vi "Stack Header (SubVI).vi"(7 "Image Size":T1={"Height"=3072, "Width"=3072}) -> (3 "Complete Header":u8[](array[numeric]))   [LabVIEW 2015]
uses:
  Controls (HOST)/Image Size.ctl
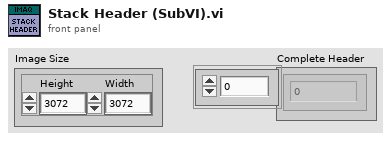
[diagram p1: front panel]
types:
  T1 = typedef "Image Size.ctl" = cluster{"Height":u16, "Width":u16}
  T2 = enum16{"big-endian, network order", "native, host order", "little-endian"}
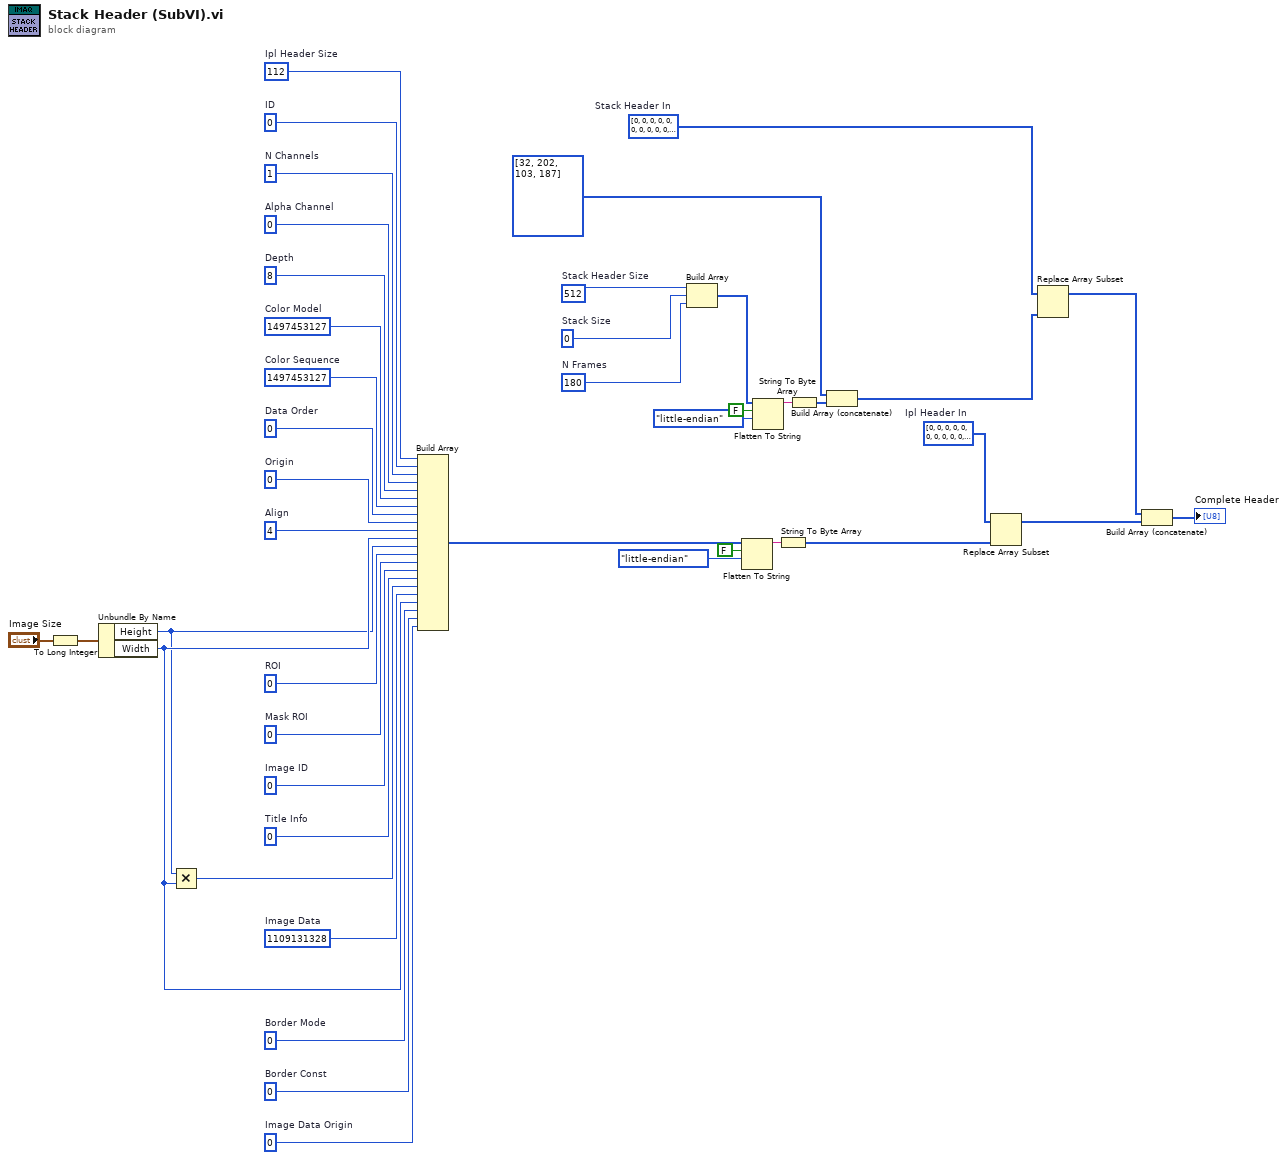
[diagram p0: block diagram]
diagram:
  w10 = 180  # N Frames
  w11 = 0  # Stack Size
  w12 = 512  # Stack Header Size
  w2 = u8[] [0, 0, 0, 0, 0, 0, 0, 0, 0, 0, 0, 0, 0, 0, 0, 0, 0, 0, 0, 0, 0, 0, 0, 0, 0, 0, 0, 0, 0, 0, 0, 0, 0, 0, 0, 0, 0, 0, 0, 0, 0, 0, 0, 0, 0, 0, 0, 0, 0, 0, 0, 0, 0, 0, 0, 0, 0, 0, 0, 0, 0, 0, 0, 0, 0, 0, 0, 0, 0, 0, 0, 0, 0, 0, 0, 0, 0, 0, 0, 0, 0, 0, 0, 0, 0, 0, 0, 0, 0, 0, 0, 0, 0, 0, 0, 0, 0, 0, 0, 0, 0, 0, 0, 0, 0, 0, 0, 0, 0, 0, 0, 0, 0, 0, 0, 0, 0, 0, 0, 0, 0, 0, 0, 0, 0, 0, 0, 0, 0, 0, 0, 0, 0, 0, 0, 0, 0, 0, 0, 0, 0, 0, 0, 0, 0, 0, 0, 0, 0, 0, 0, 0, 0, 0, 0, 0, 0, 0, 0, 0, 0, 0, 0, 0, 0, 0, 0, 0, 0, 0, 0, 0, 0, 0, 0, 0, 0, 0, 0, 0, 0, 0, 0, 0, 0, 0, 0, 0, 0, 0, 0, 0, 0, 0, 0, 0, 0, 0, 0, 0, 0, 0, 0, 0, 0, 0, 0, 0, 0, 0, 0, 0, 0, 0, 0, 0, 0, 0, 0, 0, 0, 0, 0, 0, 0, 0, 0, 0, 0, 0, 0, 0, 0, 0, 0, 0, 0, 0, 0, 0, 0, 0, 0, 0, 0, 0, 0, 0, 0, 0, 0, 0, 0, 0, 0, 0, 0, 0, 0, 0, 0, 0, 0, 0, 0, 0, 0, 0, 0, 0, 0, 0, 0, 0, 0, 0, 0, 0, 0, 0, 0, 0, 0, 0, 0, 0, 0, 0, 0, 0, 0, 0, 0, 0, 0, 0, 0, 0, 0, 0, 0, 0, 0, 0, 0, 0, 0, 0, 0, 0, 0, 0, 0, 0, 0, 0, 0, 0, 0, 0, 0, 0, 0, 0, 0, 0, 0, 0, 0, 0, 0, 0, 0, 0, 0, 0, 0, 0, 0, 0, 0, 0, 0, 0, 0, 0, 0, 0, 0, 0, 0, 0, 0, 0, 0, 0, 0, 0, 0, 0, 0, 0, 0, 0, 0, 0, 0, 0, 0, 0, 0, 0, 0, 0, 0, 0, 0, 0, 0, 0, 0, 0, 0, 0, 0, 0, 0, 0, 0, 0, 0, 0, 0, 0, 0, 0, 0, 0, 0, 0, 0, 0, 0, 0, 0, 0, 0, 0, 0, 0, 0, 0, 0, 0, 0, 0, 0, 0, 0, 0, 0, 0, 0, 0, 0, 0, 0, 0, 0, 0, 0, 0, 0, 0, 0, 0, 0, 0, 0, 0, 0, 0, 0, 0, 0, 0, 0, 0, 0, 0, 0, 0, 0, 0, 0, 0, 0, 0, 0, 0, 0, 0, 0, 0, 0, 0, 0, 0, 0, 0, 0, 0, 0, 0, 0, 0, 0, 0, 0, 0, 0, 0, 0, 0, 0, 0, 0, 0, 0, 0, 0, 0, 0, 0, 0, 0, 0, 0, 0, 0, 0, 0, 0, 0, 0, 0, 0, 0, 0, 0, 0, 0]  # Stack Header In
  w40 = u8[] [0, 0, 0, 0, 0, 0, 0, 0, 0, 0, 0, 0, 0, 0, 0, 0, 0, 0, 0, 0, 0, 0, 0, 0, 0, 0, 0, 0, 0, 0, 0, 0, 0, 0, 0, 0, 0, 0, 0, 0, 0, 0, 0, 0, 0, 0, 0, 0, 0, 0, 0, 0, 0, 0, 0, 0, 0, 0, 0, 0, 0, 0, 0, 0, 0, 0, 0, 0, 0, 0, 0, 0, 0, 0, 0, 0, 0, 0, 0, 0, 0, 0, 0, 0, 0, 0, 0, 0, 0, 0, 0, 0, 0, 0, 0, 0, 0, 0, 0, 0, 0, 0, 0, 0, 0, 0, 0, 0, 0, 0, 0, 0]  # Ipl Header In
  w39 = 112  # Ipl Header Size
  w13 = 0  # ID
  w14 = 1  # N Channels
  w15 = 0  # Alpha Channel
  w16 = 8  # Depth
  w17 = 1497453127  # Color Model
  w18 = 1497453127  # Color Sequence
  w19 = 0  # Data Order
  w20 = 0  # Origin
  w21 = 4  # Align
  w22 = 0  # ROI
  w23 = 0  # Mask ROI
  w24 = 0  # Image ID
  w25 = 0  # Title Info
  w26 = 1109131328  # Image Data
  w27 = 0  # Border Mode
  w28 = 0  # Border Const
  w29 = 0  # Image Data Origin
  n1 = To Long Integer(number="Image Size") -> (32bit integer=w31:cluster{"Height":i32, "Width":i32})
  n2 = Unbundle By Name(w31) -> ("Height"=w32:i32, "Width"=w33:i32)
  n3 = Multiply(x=w32, y=w33) -> (x*y=w34:i32)
  n4 = Build Array(w39, w13, w14, w15, w16, w17, w18, w19, w20, w21, w33, w32, w22, w23, w24, w25, w34, w26, w33, w27, w28, w29) -> (w38:i32[])
  n5 = Build Array(w12, w11, w10) -> (w6:i32[])
  n6 = Flatten To String(anything=w38, prepend array or string size? (T)=FALSE, byte order (0:big-endian, network order)=T2."little-endian") -> (data string=w35:string)  [unwired: 1 in, 2 out]
  n7 = Flatten To String(anything=w6, prepend array or string size? (T)=FALSE, byte order (0:big-endian, network order)=T2."little-endian") -> (data string=w9:string)  [unwired: 1 in, 2 out]
  n8 = String To Byte Array(string=w35) -> (unsigned byte array=w41:u8[])
  n9 = String To Byte Array(string=w9) -> (unsigned byte array=w5:u8[])
  n10 = Build Array (concatenate)(u8[] [32, 202, 103, 187] ("Image ID Code"), w5) -> (w1:u8[])
  n11 = Replace Array Subset(array=w40, new element=w41) -> (w42:u8[])  [unwired: 1 in]
  n12 = Replace Array Subset(array=w2, new element=w1) -> (w3:u8[])  [unwired: 1 in]
  n13 = Build Array (concatenate)(w3, w42) -> (→"Complete Header":u8[])
